vi "Turn.vi"(10 "Gyro":dbl format="%#_13g", 11 "Effort":dbl) -> ()   [LabVIEW 2016]
uses:
  <vilib>/Rock Robotics/WPI/SafetyOutput/WPI_SafetyOutputConfigMenu.ctl
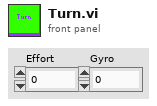
[diagram p1: front panel]
types:
  T1 = typedef "WPI_SafetyOutputConfigMenu.ctl" = enum16{"Enable", "Disable"}
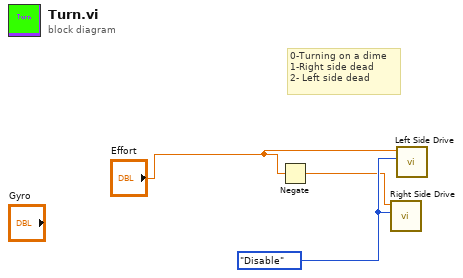
[diagram p0: block diagram]
diagram:
  w3 = WPI_SafetyOutputConfigMenu."Disable" ("mode")
  # "0-Turning on a dime\n1-Right side dead\n2- Left side dead"
  n1 = Negate(x="Effort") -> (-x=w1:dbl)
  n2 = call "Right Side Drive.vi"("mode"=w3, "Effort"=w1) -> ()  [unwired: 10 in]
  n3 = call "Left Side Drive.vi"("mode"=w3, "Effort"="Effort") -> ()  [unwired: 10 in]
